vi "TellParent.vi"(6 "Error":errorcluster, 7 "Actor":refnum<class "Actor.lvclass">, 10 "MsgDVR":refnum<data-value>, 11 "Actor":T1) -> (3 "Actor":T1, 4 "Error":errorcluster, 5 "Actor":refnum<class "Actor.lvclass">)   [LabVIEW 2020, in "jettl.lvlib"]
uses:
  jettl.lvlib
  Msg/Msg.lvclass
  Metadata/Metadata.lvclass
  Actor/Actor.lvclass
  Origin.ctl
  Msg.ctl
  PostSetup.ctl
  PreSetup.ctl
  MsgNames.ctl
  Lifecycle.ctl
  ActorAttribs.ctl
  ChildActors.ctl
  Actor.ctl
  MsgAttribs.ctl
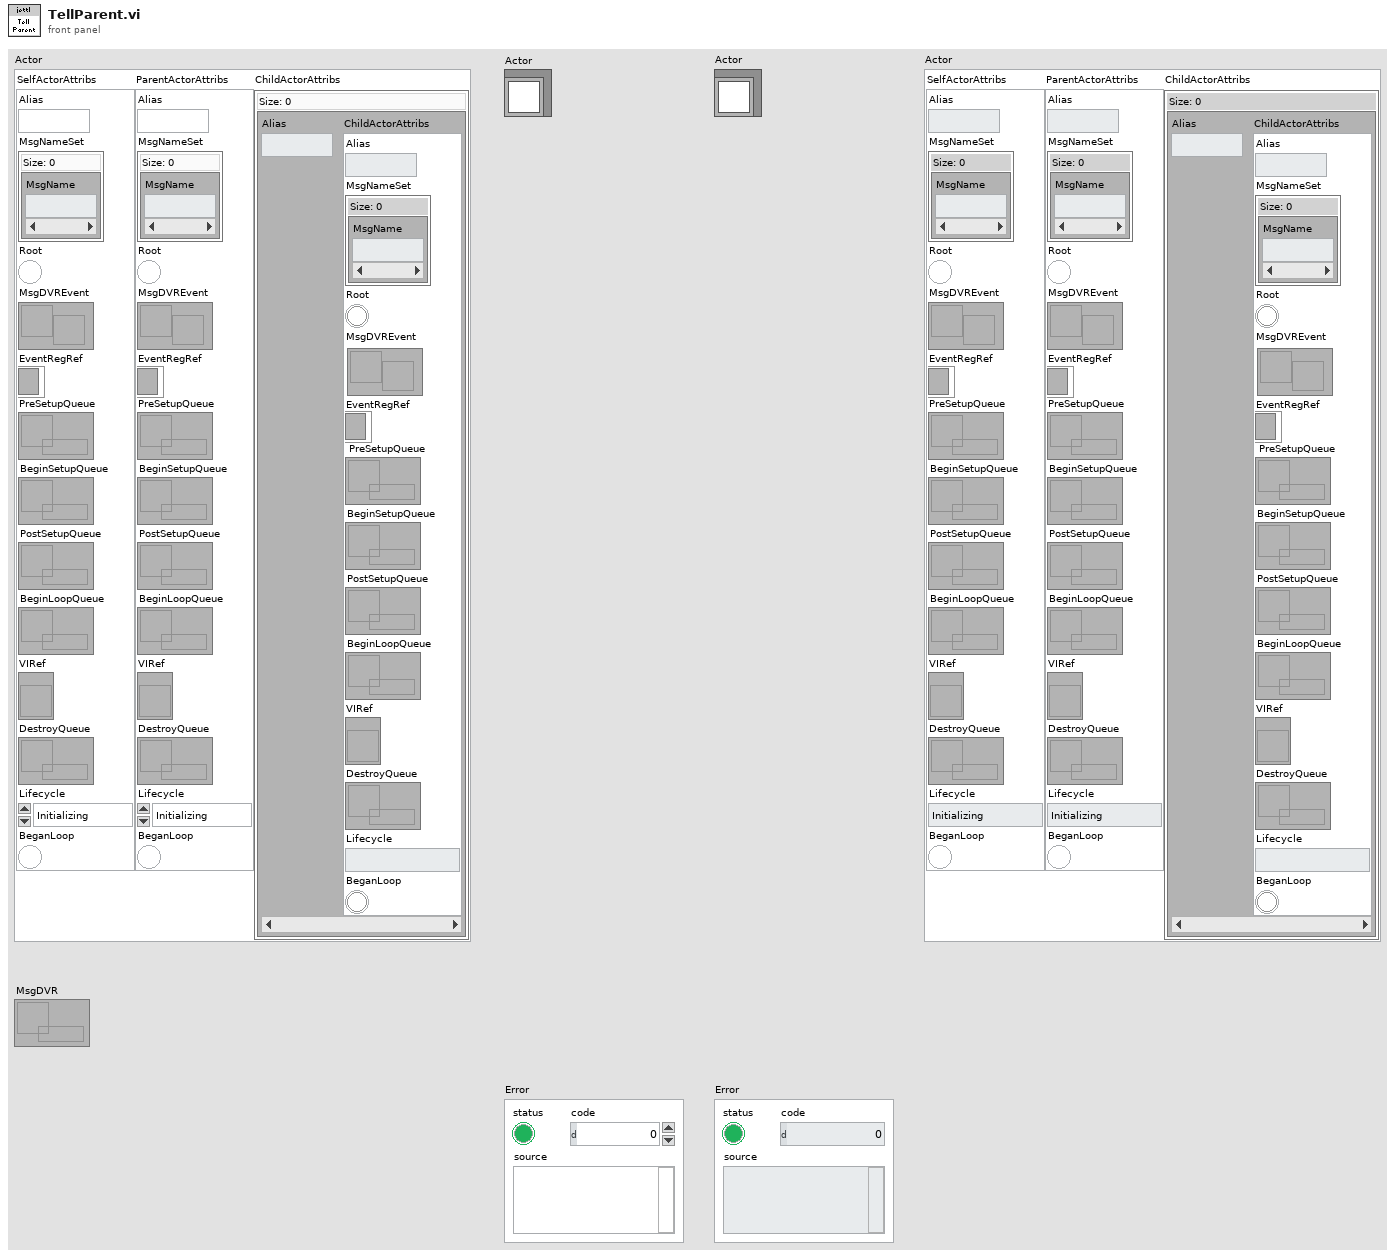
[diagram p1: front panel]
types:
  T1 = typedef "jettl.lvlib/Actor.ctl" = cluster{"SelfActorAttribs":T2, "ParentActorAttribs":T2, "ChildActorAttribs":T5}
  T2 = typedef "jettl.lvlib/ActorAttribs.ctl" = cluster{"Alias":string, "MsgNameSet":T3, "Root":bool, "MsgDVREvent":refnum<user-event>, "EventRegRef":refnum<event-registration>, "PreSetupQueue":refnum<queue>, "BeginSetupQueue":refnum<queue>, "PostSetupQueue":refnum<queue>, "BeginLoopQueue":refnum<queue>, "VIRef":refnum<vi>, "DestroyQueue":refnum<queue>, "Lifecycle":T4, "BeganLoop":bool}
  T3 = typedef "jettl.lvlib/MsgNames.ctl" = set{string}
  T4 = typedef "jettl.lvlib/Lifecycle.ctl" = enum16{"Initializing", "SettingUp", "Starting", "Running", "Stopping", "TearingDown", "Terminated"}
  T5 = typedef "jettl.lvlib/ChildActors.ctl" = map{string, T2}
  T6 = typedef "jettl.lvlib/Origin.ctl" = enum16{"Self", "Parent", "Child"}
  T7 = typedef "jettl.lvlib/PreTell.ctl" = cluster{"MsgAttribsDVR":refnum<data-value>, "Msg":refnum<class "Msg.lvclass">}
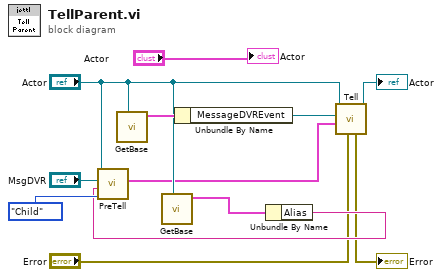
[diagram p0: block diagram]
diagram:
  n1 = call-dynamic "GetBase.vi"("Actor"="Actor") -> ("Base"=w10:T1)  [unwired: 10 in]
  n2 = call-dynamic "GetBase.vi"("Actor"="Actor") -> ("Base"=w6:T1)  [unwired: 10 in]
  n3 = Unbundle By Name(w10) -> ("MessageDVREvent"=w9:refnum<user-event>)
  n4 = Unbundle By Name(w6) -> ("Alias"=w5:string)
  n5 = call "PreTell.vi"("Origin"=Origin."Child" ("TellOrigin"), "ListenerAlias"=w5, "MsgPreTell"="MsgDVR", "ActorDVR"="Actor") -> ("MsgPreTell"=w4:T7)  [unwired: 6 in, 1 out]
  n6 = call "Tell.vi"("Error"="Error", "MsgPreTell"=w4, "MessageClusterDVREvent"=w9, "Actor"="Actor") -> ("Actor"=→"Actor":refnum<class "Actor.lvclass">, "Error"=→"Error":errorcluster)  [unwired: 6 in]
  "Actor" <- "Actor"
